vi "写入当前数值.vi"(8 "error in (no error)":errorcluster caption="错误输入（无错误）", 10 "当前数值":string, 11 "计算器类输入":refnum<class "计算器类.lvclass">) -> (0 "error out":errorcluster caption="错误输出", 3 "计算器类输出":refnum<class "计算器类.lvclass">)   [LabVIEW 2020, in "计算器类.lvclass"]
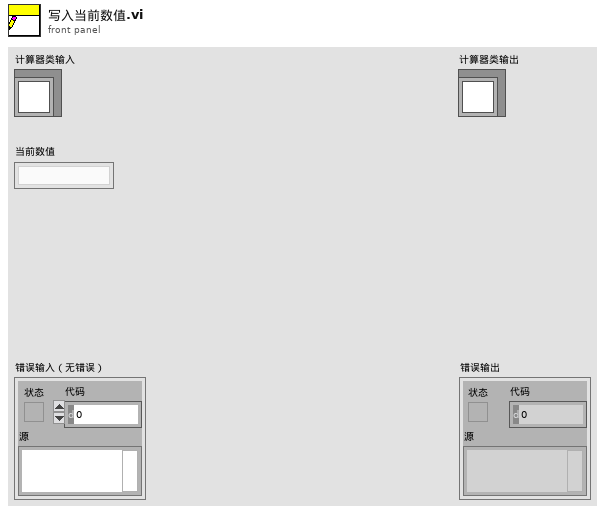
[diagram p1: front panel]
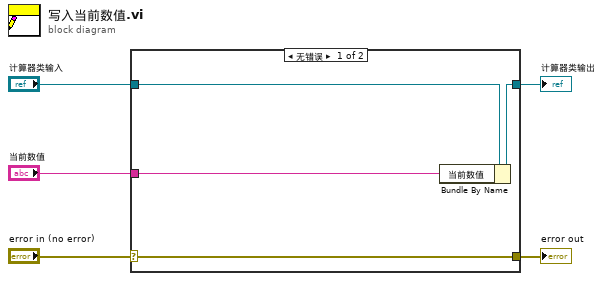
[diagram p0: block diagram]
diagram:
  n1 = case shown="无错误" "error in (no error)" {
    selector: "error in (no error)" -> [w9 w10]
    tunnel: [w9 w10] -> w4
    tunnel: [w7 w11] -> w2
    tunnel: "计算器类输入" -> [w8 w11]
    tunnel: "当前数值" -> [w6 _]
    frame No Error {
      n2 = Bundle By Name(cluster=w8, "当前数值"=w6) -> (w7:refnum<class "计算器类.lvclass">)
    }
    frame Error {
    }
  }
  "error out" <- w4
  "计算器类输出" <- w2
